vi "IBW aperture Commands.vi"(1 "input string":string="Display 'y_#wave#' vs 'x_#wave#'\nAppendToGraph 'y_#wave#' vs 'x_#wave#'\nLabel bottom \"#labelX#\"\nLabel left \"#labelY#\"\nModifyGraph rgb('y_#wave#')=(#r#,#g#,#b#)\nLegend/C/N=text0", 2 "Y label":string, 3 "X label":string, 4 "wavenames":string[](array[string])=["TEST1.5.Vx", "TEST1.5.Vy"]) -> (0 "result string":string="Display 'y_TEST1.5.Vx' vs 'x_TEST1.5.Vx'\nAppendToGraph 'y_TEST1.5.Vy' vs 'x_TEST1.5.Vy'\nLabel bottom \"bias (V)\"\nLabel left \"energyy (eV)\"\nModifyGraph rgb('y_TEST1.5.Vx')=(65280,0,0)\nModifyGraph rgb('y_TEST1.5.Vy')=(0,65280,45568)\nLegend/C/N=text0/J/X=-30.00/Y=40.00")   [LabVIEW 2016, in "LV-Data.ITX.lvclass"]
uses:
  LV-Data.ITX.lvclass
  <userlib>/LevyLab/Graph Utilities/graph_utilities.lvclass
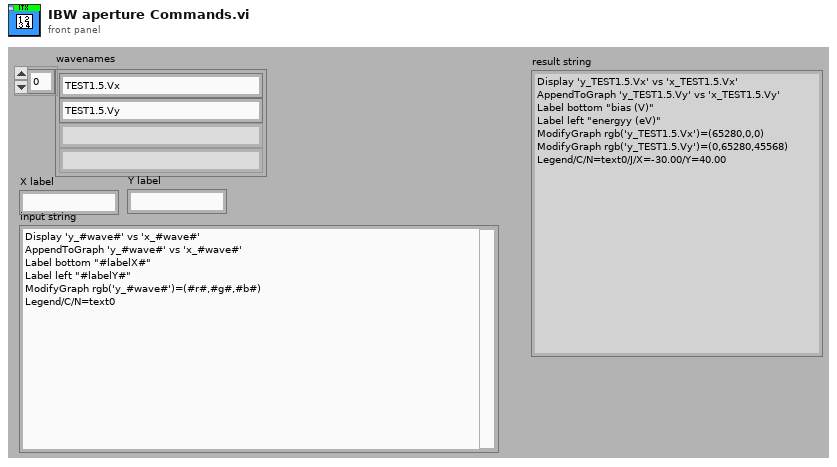
[diagram p1: front panel]
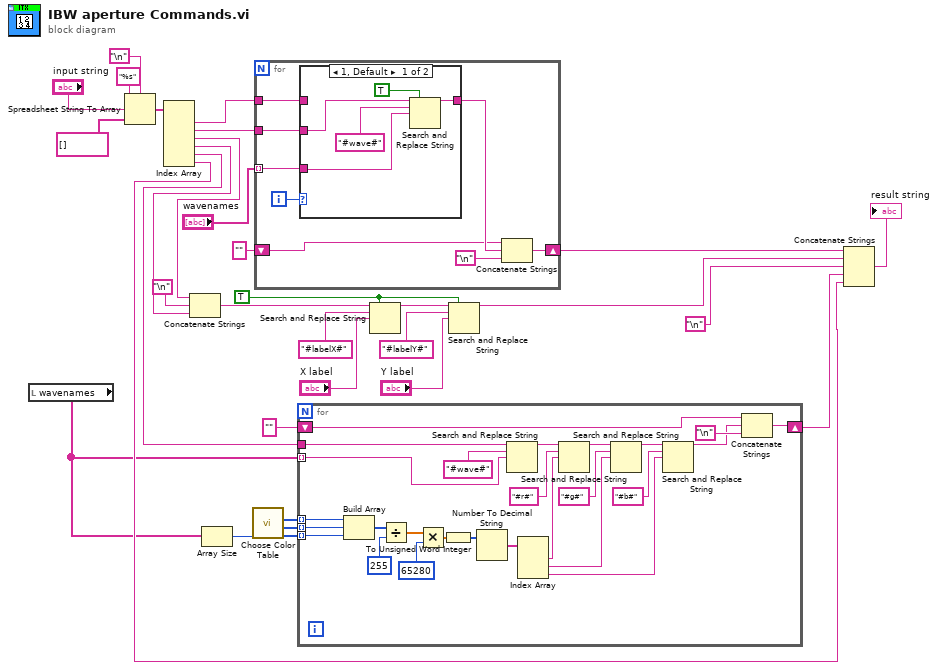
[diagram p0: block diagram]
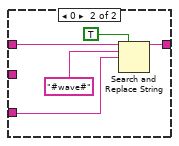
[diagram p2: hidden frame]
diagram:
  w11 = TRUE ("replace all? (F)")
  n1 = local read "wavenames"() -> (w6:string[])
  n2 = Spreadsheet String To Array(delimiter (Tab)="\n", format string="%s", spreadsheet string="input string", array type (2D Dbl)=string[] []) -> (array=w23:string[])
  n3 = Index Array(array=w23) -> (element #1=w22:string, element #2=w21:string, element #3=w18:string, element #4=w16:string, element #5=w12:string, element #6=w7:string)  [unwired: 6 in]
  n4 = Concatenate Strings(w18, "\n", w16) -> (w19:string)
  n5 = Array Size(array=w6) -> (size(s)=w5:i32)
  n6 = call <userlib>:"Choose Color Table.vi"("Size (256)"=w5) -> ("B []"=w2:u8[], "G []"=w3:u8[], "R []"=w4:u8[])  [unwired: 7 in, 1 out]
  n7 = for {
    tunnel: "wavenames" -> [w38] mode=indexing
    tunnel: w22 -> [w40]
    tunnel: w21 -> [w39]
    shift-right: [w36] -> w27
    shift-left: "" -> [w33]
    i -> [w37]
    n8 = case shown="1, Default" w37 {
      tunnel: w40 -> [_ w48]
      tunnel: w39 -> [w43 _]
      tunnel: w38 -> [w44 w49]
      tunnel: [w42 w47] -> w35
      frame 1, Default {
        n9 = Search and Replace String(replace all?=TRUE ("replace all? (F)"), input string=w43, search string="#wave#", replace string=w44) -> (result string=w42:string)  [unwired: 1 in, 6 out]
      }
      frame 0 {
        n10 = Search and Replace String(replace all?=TRUE ("replace all? (F)"), input string=w48, search string="#wave#", replace string=w49) -> (result string=w47:string)  [unwired: 1 in, 6 out]
      }
    }
    n11 = Concatenate Strings(w33, w35, "\n") -> (w36:string)
  }
  n12 = for {
    tunnel: w12 -> [w69]
    tunnel: w6 -> [w51] mode=indexing
    shift-right: [w65] -> w1
    shift-left: "" -> [w64]
    tunnel: w4 -> [w54] mode=indexing
    tunnel: w3 -> [w53] mode=indexing
    tunnel: w2 -> [w52] mode=indexing
    n13 = Build Array(w54, w53, w52) -> (w76:u8[])
    n14 = Divide(x=w76, y=255) -> (x/y=w72:dbl[])
    n15 = Multiply(x=w72, y=65280) -> (x*y=w73:dbl[])
    n16 = To Unsigned Word Integer(number=w73) -> (unsigned 16bit integer=w71:u16[])
    n17 = Number To Decimal String(number=w71) -> (decimal integer string=w58:string[])  [unwired: 1 out]
    n18 = Search and Replace String(input string=w69, search string="#wave#", replace string=w51) -> (result string=w70:string)  [unwired: 1 in, 7 out]
    n19 = Index Array(array=w58) -> (element #1=w57:string, element #2=w56:string, element #3=w55:string)  [unwired: 3 in]
    n20 = Search and Replace String(input string=w70, search string="#r#", replace string=w57) -> (result string=w68:string)  [unwired: 1 in, 7 out]
    n21 = Search and Replace String(input string=w68, search string="#g#", replace string=w56) -> (result string=w67:string)  [unwired: 1 in, 7 out]
    n22 = Search and Replace String(input string=w67, search string="#b#", replace string=w55) -> (result string=w62:string)  [unwired: 1 in, 7 out]
    n23 = Concatenate Strings(w64, w62, "\n") -> (w65:string)
  }
  n24 = Search and Replace String(replace all?=w11, input string=w19, search string="#labelX#", replace string="X label") -> (result string=w15:string)  [unwired: 1 in, 6 out]
  n25 = Search and Replace String(replace all?=w11, input string=w15, search string="#labelY#", replace string="Y label") -> (result string=w9:string)  [unwired: 1 in, 6 out]
  n26 = Concatenate Strings(w27, w9, "\n", w1, w7) -> (→"result string":string)
